vi "Polling Start Core.vi"(8 "Error In":errorcluster, 11 "BNT_DAQmx-MCSV-DOPWM in":refnum<class "BNT_DAQmx-MCSV-DOPWM.lvclass">) -> (0 "Error Out":errorcluster, 3 "BNT_DAQmx-MCSV-DOPWM out":refnum<class "BNT_DAQmx-MCSV-DOPWM.lvclass">)   [LabVIEW 2019, in "BNT_DAQmx.lvlib" / "BNT_DAQmx-MCSV-DOPWM.lvclass"]
doc: "Implement your code to start polling here."
uses:
  BNT_DAQmx-MCSV-DOPWM.lvclass
  BNT_DAQmx-MCSV-DOPWM.lvclass/BNT_DAQmx-MCSV-DOPWM.ctl
  BNT_DAQmx-MCSV/BNT_DAQmx-MCSV.lvclass
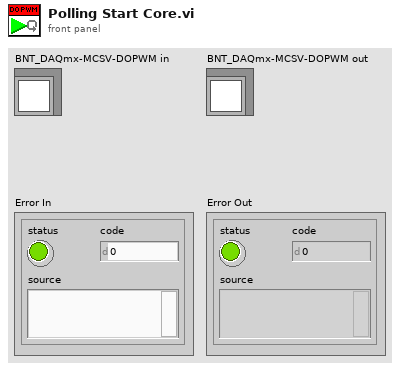
[diagram p1: front panel]
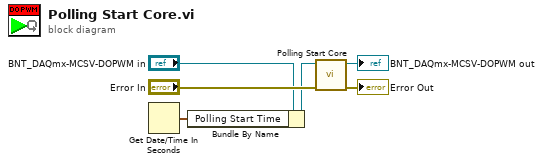
[diagram p0: block diagram]
diagram:
  n1 = Get Date/Time In Seconds() -> (seconds since 1Jan1904=w1:timestamp)
  n2 = Bundle By Name(cluster="BNT_DAQmx-MCSV-DOPWM in", "Polling Start Time"=w1) -> (w2:refnum<class "BNT_DAQmx-MCSV-DOPWM.lvclass">)
  n3 = call-parent "Polling Start Core.vi"("Error In"="Error In", "CSPP_BaseActor in"=w2) -> ("Error Out"=→"Error Out":errorcluster, "CSPP_BaseActor out"=→"BNT_DAQmx-MCSV-DOPWM out":refnum<class "BNT_DAQmx-MCSV-DOPWM.lvclass">)  [unwired: 8 in]
